vi "Print Debug Line.vi"(6 "Append newline? (T)":bool=TRUE, 7 "Add to log file? (F)":bool, 8 "error in":errorcluster, 10 "Message":string, 11 "NIVS Custom Device API in":refnum<class "NIVS Custom Device API.lvclass">) -> (0 "error out":errorcluster, 3 "NIVS Custom Device API out":refnum<class "NIVS Custom Device API.lvclass">)   [LabVIEW 2026, in "NIDMM Engine.lvlib" / "NIVS Custom Device API.lvclass"]
uses:
  NIVS Custom Device API.lvclass
  NIVS Custom Device API.lvclass/NIVS Custom Device API.ctl
  <vilib>/NI VeriStand/Custom Device Tools/Custom Device Utility Library/Custom Device Utility Library.lvlib
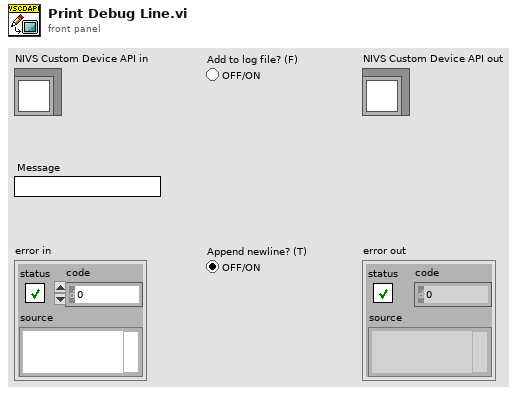
[diagram p1: front panel]
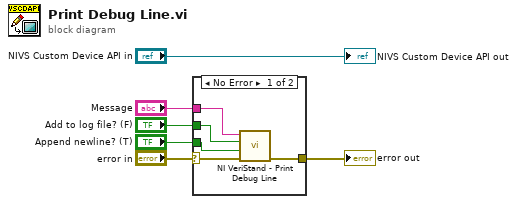
[diagram p0: block diagram]
diagram:
  n1 = case shown="No Error" "error in" {
    selector: "error in" -> [w11 w12]
    tunnel: [w10 w12] -> w4
    tunnel: "Message" -> [w9 _]
    tunnel: "Add to log file? (F)" -> [w8 _]
    tunnel: "Append newline? (T)" -> [w7 _]
    frame No Error {
      n2 = call <vilib>:"NI VeriStand - Print Debug Line.vi"("error in (no error)"=w11, "Append newline? (T)"=w7, "Add to log file? (F)"=w8, "Message"=w9) -> ("error out"=w10:errorcluster)  [unwired: 7 in]
    }
    frame Error {
    }
  }
  "error out" <- w4
  "NIVS Custom Device API out" <- "NIVS Custom Device API in"
